vi "Test Ultrasonic Sensor.vi"() -> ()   [LabVIEW 2012]
uses:
  <vilib>/robotics/Starter Kit/2.0/9632 Host Interface/NI_Robotics_Starter Kit Host_9632_2.0.lvclass
  <vilib>/robotics/Starter Kit/Host Interface/NI_Robotics_Starter Kit Host.lvclass
panel:
  out "Sensor Distance (m)":dbl(graph)
  out "Object Detected":bool
  in  "stop":bool
  # "Move in front of the ultrasonic sensor to confirm that it can detect objects."
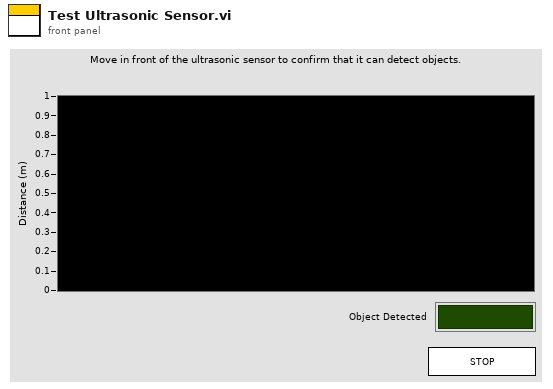
[diagram p1: front panel]
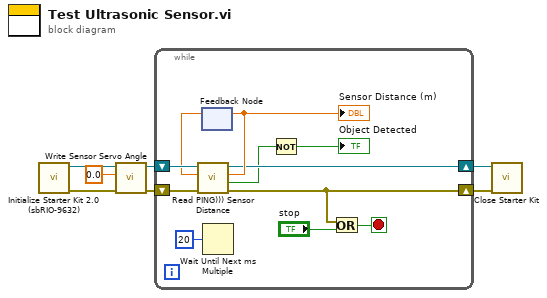
[diagram p0: block diagram]
diagram:
  n1 = call <vilib>:"Initialize Starter Kit 2.0 (sbRIO-9632).vi"() -> ("error out"=w3:errorcluster, "FPGA starter kit host 2.0 out"=w4:refnum<class "NI_Robotics_Starter Kit Host_9632_2.0.lvclass">)  [unwired: 10 in]
  n2 = call <vilib>:"Write Sensor Servo Angle.vi"("error in (no error)"=w3, "ccw servo angle (rad)"=0.0 ("sensor motor angle (rad)"), "starter kit host in"=w4) -> ("error out"=w1:errorcluster, "starter kit host out"=w2:refnum<class "NI_Robotics_Starter Kit Host_9632_2.0.lvclass">)  [unwired: 7 in]
  n3 = while {
    shift-right: [w13] -> w7
    shift-left: w2 -> [w11]
    shift-right: [w8] -> w6
    shift-left: w1 -> [w10]
    stop <- w17 stop-if-true
    n4 = feedback #1() -> (w9:dbl)  [unwired: 1 in]
    n5 = call <vilib>:"Read PING))) Sensor Distance.vi"("error in (no error)"=w10, "default distance (NaN)"=w9, "starter kit host in"=w11) -> ("error out"=w8:errorcluster, "timed out?"=w12:bool, "distance (m)"=w14:dbl, "starter kit host out"=w13:refnum<class "NI_Robotics_Starter Kit Host_9632_2.0.lvclass">)  [unwired: 5 in]
    "Sensor Distance (m)" <- w14
    n6 = feedback-in #1(w14) -> ()
    n7 = Wait Until Next ms Multiple(millisecond multiple=u32 20) -> ()  [unwired: 1 out]
    n8 = Not(x=w12) -> (.not. x?=→"Object Detected":bool)
    n9 = Or(x=w8, y="stop") -> (x .or. y?=w17:bool)
  }
  n10 = call-dynamic "Close Starter Kit.vi"("error in (no error)"=w6, "starter kit host in"=w7) -> ()  [unwired: 9 in, 1 out]
